vi "Autunomous Set Target.vi"() -> ()   [LabVIEW 2009]
uses:
  <vilib>/Platform/TimedLoop/XDataNode/XDataNode.xnode
  <vilib>/Platform/TimedLoop/XDataNode/loadlvalarms.vi
  <vilib>/Platform/TimedLoop/XDataNode/timing_clust.ctl
  <vilib>/Platform/TimedLoop/XDataNode/nitl_modes.ctl
  <vilib>/Platform/TimedLoop/XDataNode/wakeup.ctl
  TypeDefs/State Machine/Main State.ctl
  Functional Global Variables/Actions for FG's.ctl
  TypeDefs/Sensor TypeDefs/GPS Data.ctl
  <vilib>/Platform/TimedLoop/XDataNode/XDNodeRunTimeDep.lvlib
  <vilib>/Analysis/NI_AALBase.lvlib
  <vilib>/Analysis/NI_AALPro.lvlib
panel:
  in  "Buffer Size (Seconds)":i32=15
  in  "Path history enabled?":bool=TRUE
  in  "Buffer Dimension":i32=10
  out "Target Bearing":dbl
  in  "Prediction Time (s)":dbl=1.0
  out "XY Graph":cluster{dbl[], dbl[]}(graph)
  in  "Sampling Time":dbl[](array[numeric])
  in  "Bearing History":dbl[](array[numeric])
  out "Bearing Sample":dbl=191.29579607174375 format="%0.2f"
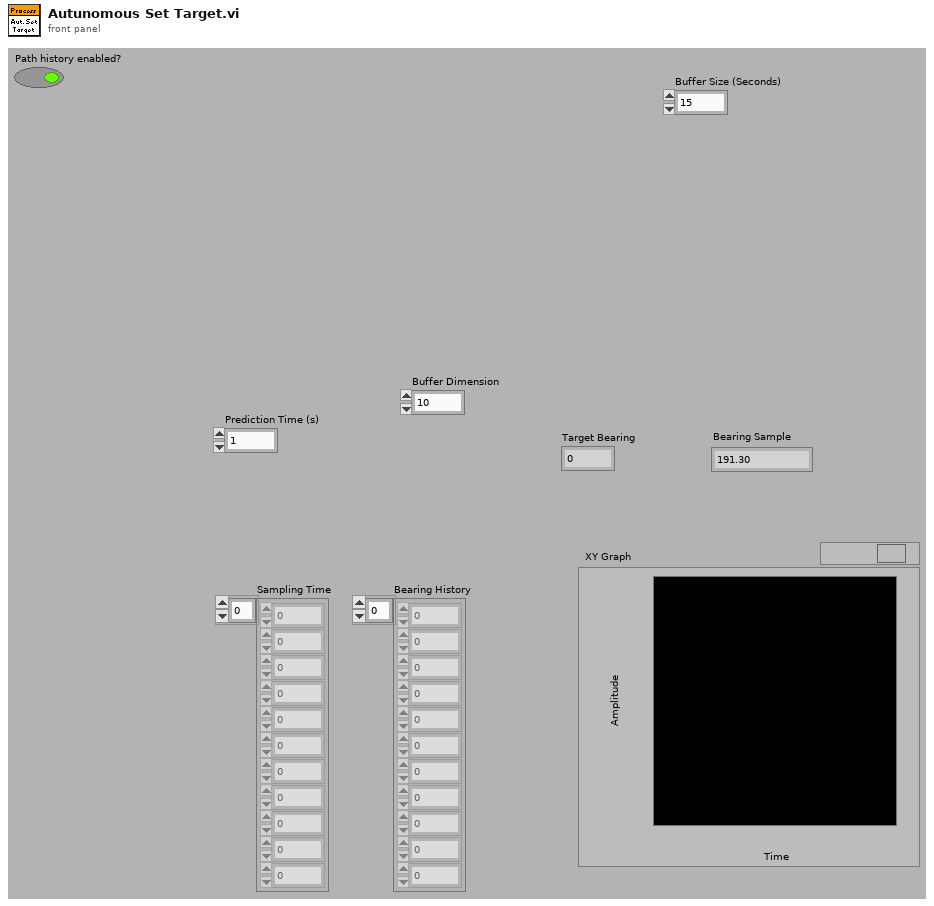
[diagram p1: front panel]
types:
  T1 = typedef "Actions for FG's.ctl" = enum16{"Read", "Write"}
  T2 = typedef "XDNodeRunTimeDep.lvlib/timing_clust.ctl" = cluster{"Expected End [f-1]":u64, "Actual End [f-1]":u64, "Finished Late? [f-1]":bool, "Expected End [i-1]":u64, "Actual End [i-1]":u64, "Finished Late? [i-1]":bool, "Expected Start [i]":u64, "Actual Start [i]":u64, "Expected Start [f]":u64, "Actual Start [f]":u64, "Source Name":string, "Structure Name":string, "Period":i64, "Deadline":i64, "Offset":i64, "Start":i64, "Priority":i32, "Timeout":i32, "Mode":T3, "Wakeup Reason":T4, "Error":errorcluster, "Source Type":string, "Secondary Source Type":string, "Global End Time":u64, "Global Start Time":u64, "Frame Duration":u64, "Iteration Duration":u64, "Assigned CPU":i32, "I/O Scan Engine Mode":u32}
  T3 = typedef "XDNodeRunTimeDep.lvlib/nitl_modes.ctl" = enum32{"No Change", "Process missed periods, maintain original phase", "Discard missed periods, maintain original phase", "Process missed periods, ignore original phase", "Discard missed periods, ignore original phase"}
  T4 = typedef "XDNodeRunTimeDep.lvlib/wakeup.ctl" = enum32{"Normal", "Aborted", "Asynchronous wakeup", "Timing source error", "Timed loop error", "Timeout"}
  T5 = typedef "Main State.ctl" = enum16{"Startup", "Wait for Init", "Initialize Sensors", "Wait for Saftey Disable", "Check Saftey", "Wait for GO", "Run", "Remote Control", "Stop"}
  T6 = typedef "GPS Data.ctl" = cluster{"Latitude":dbl, "Longitude":dbl}
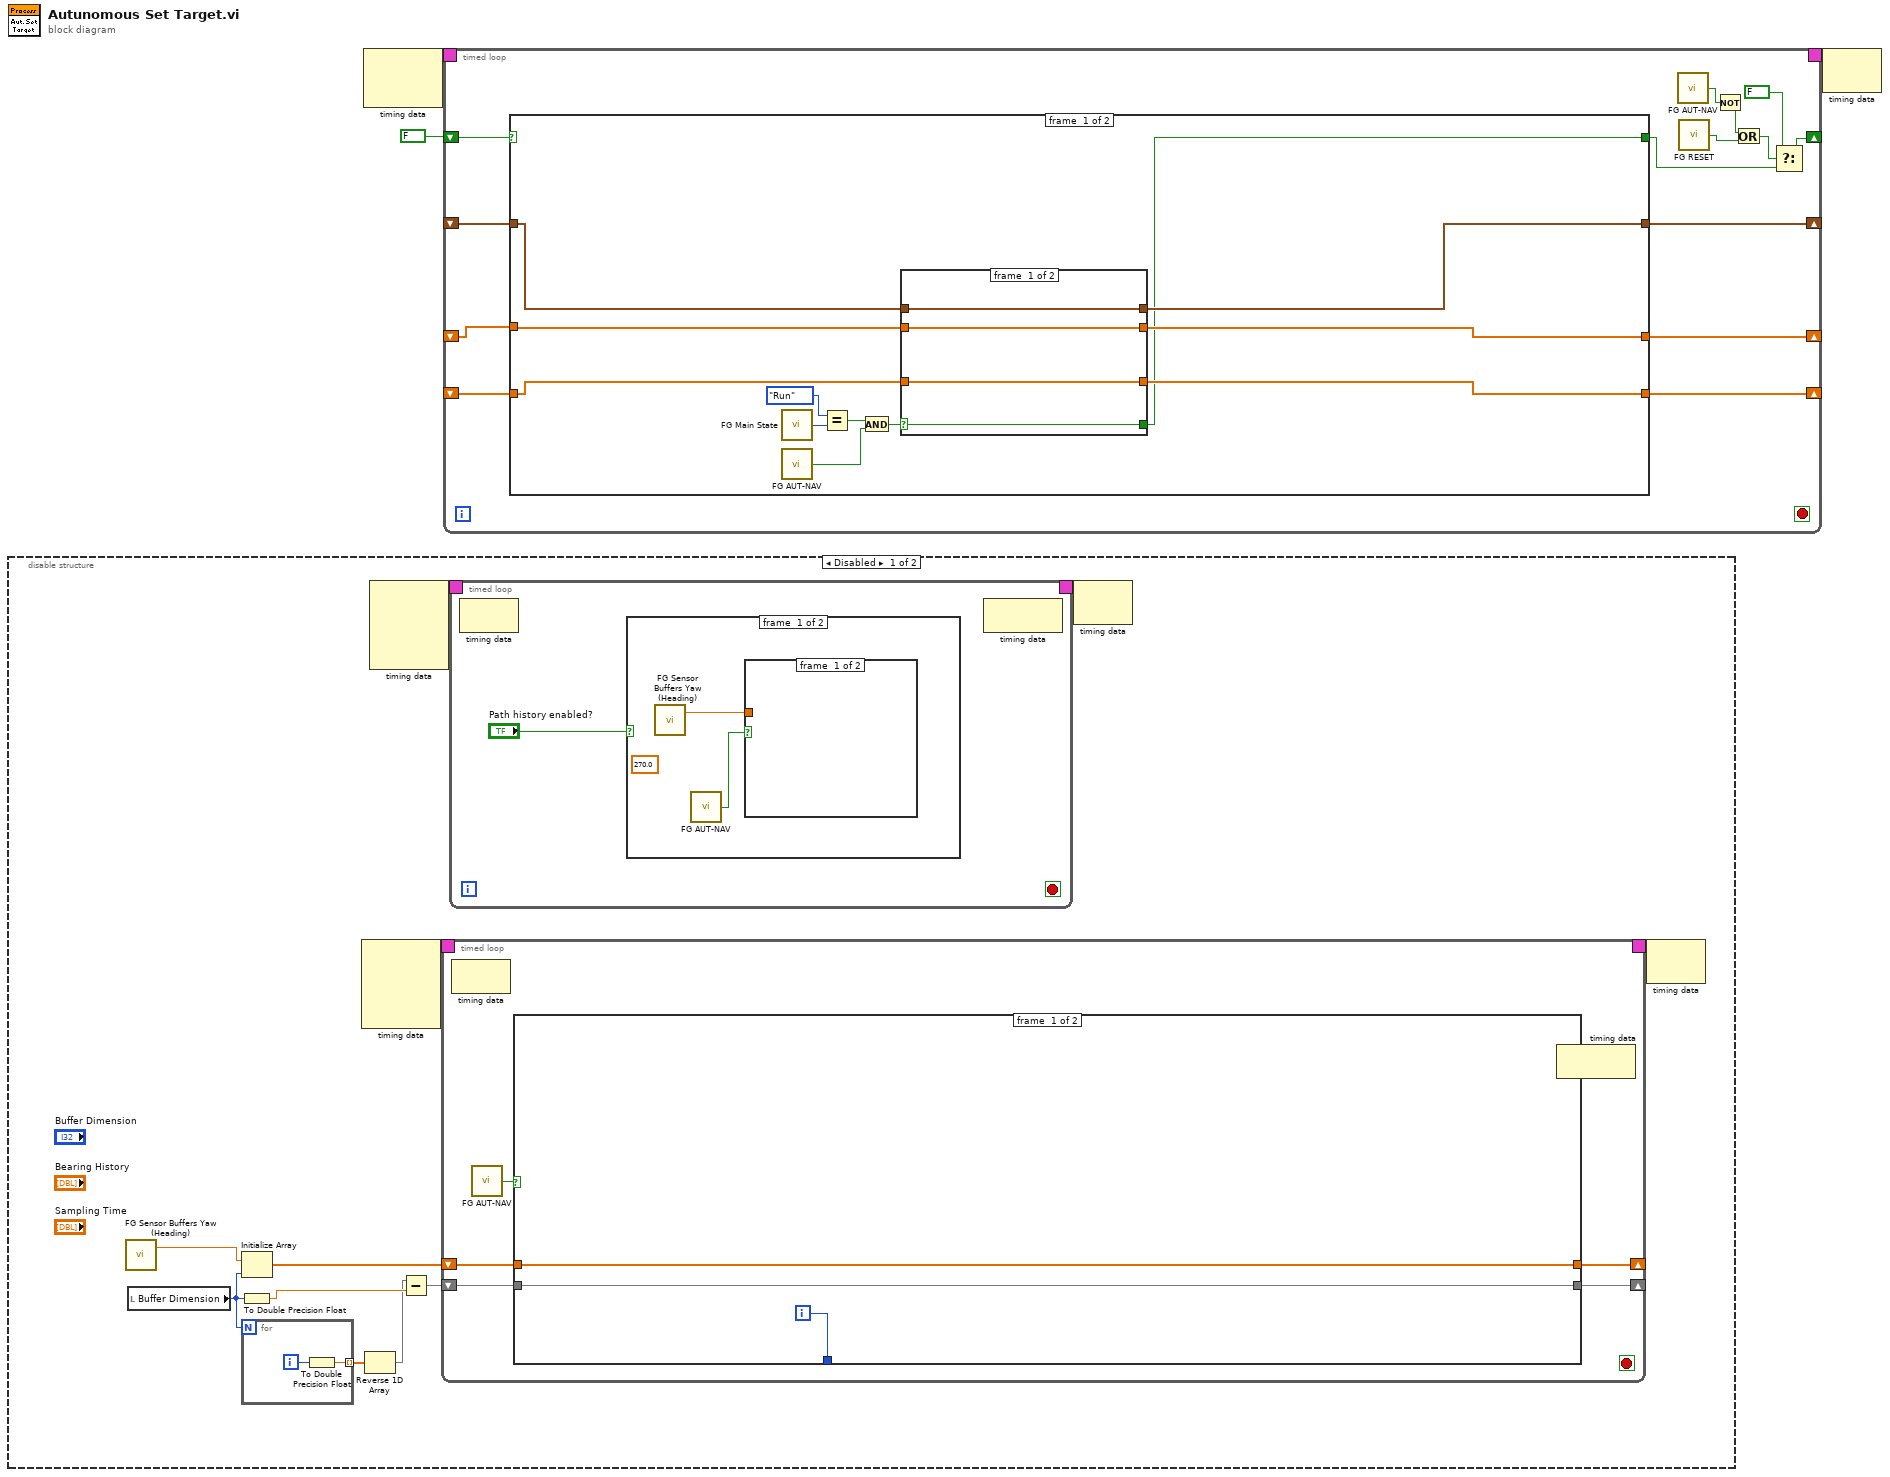
[diagram p0: block diagram]
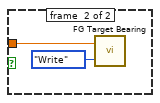
[diagram p2: hidden frame]
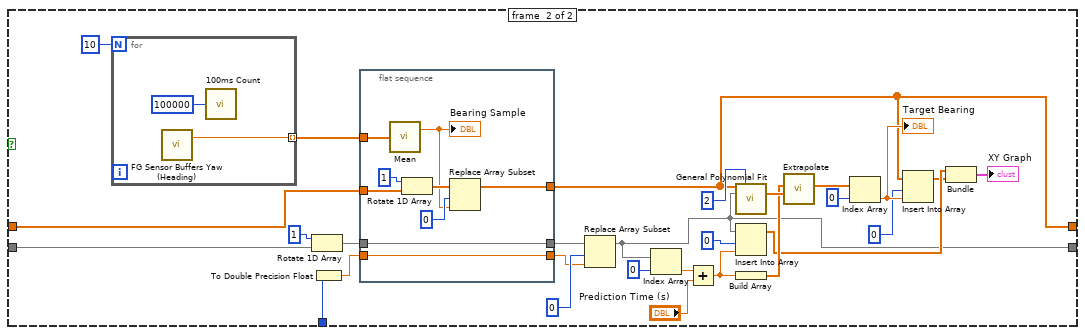
[diagram p4: hidden frame]
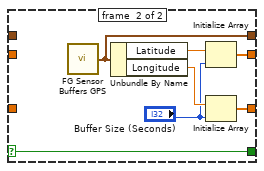
[diagram p6: hidden frame]
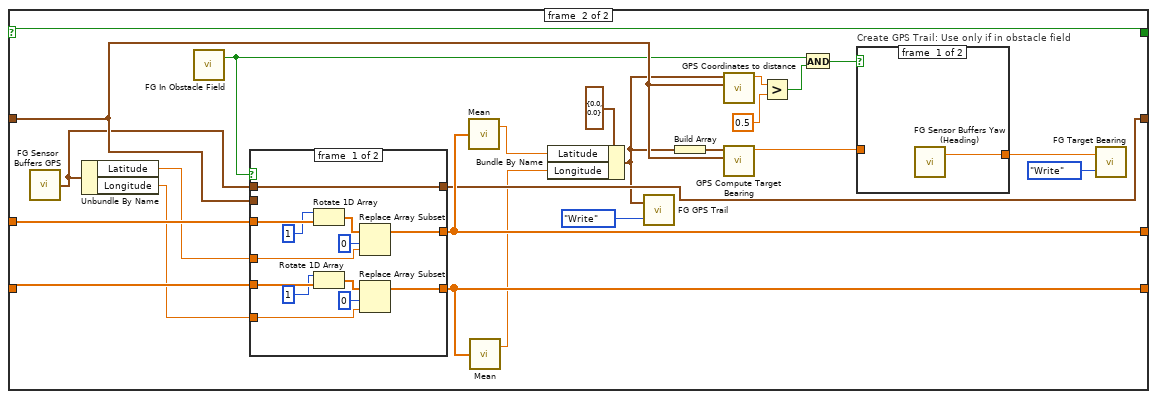
[diagram p7: hidden frame]
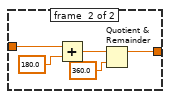
[diagram p8: hidden frame]
diagram:
  n1 = disable-structure shown="Disabled" {
    frame #0 {
      n2 = call "FG Sensor Buffers Yaw (Heading).vi"() -> ("Yaw Buffer Out"=w10:dbl)  [unwired: 3 in]
      n3 = local read "Buffer Dimension"() -> (w7:i32)
      n4 = Initialize Array(w10, w7) -> (w9:dbl[])
      n5 = To Double Precision Float(number=w7) -> (double precision float=w5:dbl)
      n6 = for {
        N: w7 -> [_]
        tunnel: [w24] -> w8 mode=indexing
        i -> [w25]
        n7 = To Double Precision Float(number=w25) -> (double precision float=w24:dbl)
      }
      n8 = node-c288() -> (w14:T2)  [unwired: 4 in]
      n9 = Reverse 1D Array(array=w8) -> (reversed array=w4:dbl[])
      n10 = node-c288() -> (w12:T2)  [unwired: 4 in]
      n11 = Subtract(x=w4, y=w5) -> (x-y=w6:dbl[])
      n12 = timed-loop {
        timing: w14 -> [_]
        timing-out: [_] -> w13
        shift-right: [w28] -> _
        shift-left: w9 -> [w29]
        shift-right: [w27] -> _
        shift-left: w6 -> [w30]
        i -> [w31]
        stop <- _ stop-if-true
        n13 = node-c288() -> ()  [unwired: 1 in, 1 out]
        n14 = call "FG AUT-NAV.vi"() -> ("Aut/!Nav out"=w26:bool)  [unwired: 2 in]
        n15 = case shown="True" w26 {
          tunnel: w31 -> [_ w59]
          tunnel: w30 -> [w32 w58]
          tunnel: w29 -> [w33 w51]
          tunnel: [w33 w35] -> w28
          tunnel: [w32 w34] -> w27
          frame #0 {
          }
          frame #1 {
            n16 = for {
              N: 10 -> [_]
              tunnel: [w72] -> w60 mode=indexing
              n17 = call "FG Sensor Buffers Yaw (Heading).vi"() -> ("Yaw Buffer Out"=w72:dbl)  [unwired: 3 in]
              n18 = call "100ms Count"("Count(uSec)"=u32 100000) -> ()  [unwired: 1 out]
            }
            n19 = Rotate 1D Array(1:w58, 2:1 ("n")) -> (0:w56:dbl[])
            n20 = To Double Precision Float(number=w59) -> (double precision float=w55:dbl)
            n21 = flat-sequence {
              tunnel: w60 -> [w70]
              tunnel: w56 -> [w69]
              tunnel: w55 -> [w68]
              tunnel: [w69] -> w53
              tunnel: [w68] -> w52
              tunnel: w51 -> [w66]
              tunnel: [w63] -> w35
              frame #0 {
                n22 = call <vilib>:"Mean.vi"("X"=w70) -> ("mean"=w62:dbl)  [unwired: 1 out]
                "Bearing Sample" <- w62
                n23 = Rotate 1D Array(1:w66, 2:1 ("n")) -> (0:w64:dbl[])
                n24 = Replace Array Subset(array=w64, new element=w62, index=0) -> (w63:dbl[])
              }
            }
            n25 = Replace Array Subset(array=w53, new element=w52, index=0) -> (w34:dbl[])
            n26 = Index Array(array=w34, index=0) -> (element=w46:dbl)
            n27 = Add(x=w46, y="Prediction Time (s)") -> (x+y=w40:dbl)
            n28 = call <vilib>:"General Polynomial Fit.vi"("Y"=w35, "polynomial order"=2, "X"=w34) -> ("Polynomial Coefficients"=w49:dbl[])  [unwired: 9 in, 3 out]
            n29 = Insert Into Array(array=w34, index=0, new element=w40) -> (w39:dbl[])
            n30 = Build Array(w40) -> (w41:dbl[])
            n31 = call "Extrapolate.vi"("Polynomial Coefficients"=w49, "xi"=w41) -> ("yi"=w48:dbl[])  [unwired: 9 in]
            n32 = Index Array(array=w48, index=0) -> (element=w42:dbl)
            "Target Bearing" <- w42
            n33 = Insert Into Array(array=w35, index=0, new element=w42) -> (w38:dbl[])
            n34 = Bundle(w39, w38) -> (→"XY Graph":cluster{dbl[], dbl[]})  [unwired: 1 in]
          }
        }
        n35 = node-c288() -> ()  [unwired: 1 in, 1 out]
      }
      n36 = timed-loop {
        timing: w12 -> [_]
        timing-out: [_] -> w11
        stop <- _ stop-if-true
        n37 = node-c288() -> ()  [unwired: 1 in, 1 out]
        n38 = case shown="False" "Path history enabled?" {
          frame #0 {
            (unwired) 270.0 ("Target Bearing in")
            n39 = call "FG Sensor Buffers Yaw (Heading).vi"() -> ("Yaw Buffer Out"=w17:dbl)  [unwired: 3 in]
            n40 = call "FG AUT-NAV.vi"() -> ("Aut/!Nav out"=w16:bool)  [unwired: 2 in]
            n41 = case shown="True" w16 {
              tunnel: w17 -> [_ w18]
              frame #0 {
              }
              frame #1 {
                n42 = call "FG Target Bearing.vi"("FG Action (Read)"=Actions_for_FG's."Write", "Target Bearing in"=w18) -> ()  [unwired: 1 out]
              }
            }
          }
          frame #1 {
          }
        }
        n43 = node-c288() -> ()  [unwired: 1 in, 1 out]
      }
      n44 = node-c288(w11) -> ()  [unwired: 1 out]
      n45 = node-c288(w13) -> ()  [unwired: 1 out]
    }
    frame #1 {
    }
  }
  n46 = node-c288() -> (w3:T2)  [unwired: 2 in]
  n47 = timed-loop {
    timing: w3 -> [_]
    timing-out: [_] -> w2
    shift-right: [w88] -> _
    shift-left: _ -> [w90]
    shift-right: [w87] -> _
    shift-left: _ -> [w89]
    shift-right: [w85] -> _
    shift-left: _ -> [w86]
    shift-right: [w82] -> _
    shift-left: FALSE ("t") -> [w84]
    stop <- _ stop-if-true
    n48 = case shown="False" w84 {
      selector: w84 -> [_ w115]
      tunnel: w90 -> [w93 w137]
      tunnel: w89 -> [w92 w136]
      tunnel: [w97 w135] -> w88
      tunnel: [w96 w134] -> w87
      tunnel: w86 -> [w94 w133]
      tunnel: [w95 w132] -> w85
      tunnel: [w91 w115] -> w81
      frame #0 {
        n49 = call "FG Main State.vi"() -> ("Main State out"=w102:T5)  [unwired: 2 in]
        n50 = call "FG AUT-NAV.vi"() -> ("Aut/!Nav out"=w98:bool)  [unwired: 2 in]
        n51 = Equal?(x=Main_State."Run" ("Main State out"), y=w102) -> (x = y?=w100:bool)
        n52 = And(x=w100, y=w98) -> (x .and. y?=w99:bool)
        n53 = case shown="False" w99 {
          selector: w99 -> [w103 w108]
          tunnel: [w105 w111] -> w97
          tunnel: [w104 w110] -> w96
          tunnel: [w106 w109] -> w95
          tunnel: w94 -> [w106 _]
          tunnel: w93 -> [w105 _]
          tunnel: w92 -> [w104 _]
          tunnel: [w103 w108] -> w91
          frame #0 {
          }
          frame #1 {
            n54 = call "FG Sensor Buffers GPS.vi"() -> ("GPS Buffer out"=w109:T6)  [unwired: 2 in]
            n55 = Unbundle By Name(w109) -> ("Latitude"=w112:dbl, "Longitude"=w113:dbl)
            n56 = Initialize Array(w112, "Buffer Size (Seconds)") -> (w111:dbl[])
            n57 = Initialize Array(w113, "Buffer Size (Seconds)") -> (w110:dbl[])
          }
        }
      }
      frame #1 {
        n58 = call "FG Sensor Buffers GPS.vi"() -> ("GPS Buffer out"=w123:T6)  [unwired: 2 in]
        n59 = Unbundle By Name(w123) -> ("Latitude"=w131:dbl, "Longitude"=w130:dbl)
        n60 = call "FG In Obstacle Field.vi"() -> ("In Obs. Field? out"=w116:bool)  [unwired: 3 in]
        n61 = case shown="False" w116 {
          tunnel: w137 -> [w156 w158]
          tunnel: w136 -> [w155 w157]
          tunnel: w131 -> [w154 _]
          tunnel: w130 -> [w153 _]
          tunnel: [w146 w158] -> w135
          tunnel: [w145 w157] -> w134
          tunnel: w123 -> [w144 _]
          tunnel: [w144 w159] -> w132
          tunnel: w133 -> [_ w159]
          frame #0 {
            n62 = Rotate 1D Array(1:w156, 2:1 ("n")) -> (0:w150:dbl[])
            n63 = Rotate 1D Array(1:w155, 2:1 ("n")) -> (0:w149:dbl[])
            n64 = Replace Array Subset(array=w150, new element=w154, index=0) -> (w146:dbl[])
            n65 = Replace Array Subset(array=w149, new element=w153, index=0) -> (w145:dbl[])
          }
          frame #1 {
          }
        }
        n66 = call <vilib>:"Mean.vi"("X"=w135) -> ("mean"=w128:dbl)  [unwired: 1 out]
        n67 = call <vilib>:"Mean.vi"("X"=w134) -> ("mean"=w124:dbl)  [unwired: 1 out]
        n68 = Bundle By Name(cluster=T6 {"Latitude"=0.0, "Longitude"=0.0} ("GPS Buffer out"), "Latitude"=w128, "Longitude"=w124) -> (w119:T6)
        n69 = call "FG GPS Trail.vi"("FG Action (Read)"=Actions_for_FG's."Write", "GPS Buffer in"=w119) -> ()  [unwired: 1 in, 1 out]
        n70 = Build Array(w119) -> (w126:T6[])
        n71 = call "GPS Coordinates to distance.vi"("GPS Co-ordinate 2"=w133, "GPS Co-ordinate 1"=w119) -> ("Distance"=w118:dbl)  [unwired: 9 in]
        n72 = call "GPS Compute Target Bearing.vi"("Current co-ordinates"=w133, "GPS Waypoint List Out"=w126) -> ("Target Bearing (degrees)"=w125:dbl)  [unwired: 8 in]
        n73 = Greater?(x=w118, y=0.5) -> (0:w120:bool)
        n74 = And(x=w116, y=w120) -> (x .and. y?=w114:bool)
        n75 = case "Create GPS Trail: Use only if in obstacle field" shown="True" w114 {
          tunnel: w125 -> [_ w143]
          tunnel: [w138 w142] -> w121
          frame #0 {
            n76 = call "FG Sensor Buffers Yaw (Heading).vi"() -> ("Yaw Buffer Out"=w138:dbl)  [unwired: 3 in]
          }
          frame #1 {
            n77 = Add(x=w143, y=180.0) -> (x+y=w140:dbl)
            n78 = Quotient & Remainder(x=w140, y=360.0) -> (x-y*floor(x/y)=w142:dbl)  [unwired: 1 out]
          }
        }
        n79 = call "FG Target Bearing.vi"("FG Action (Read)"=Actions_for_FG's."Write", "Target Bearing in"=w121) -> ()  [unwired: 1 out]
      }
    }
    n80 = call "FG AUT-NAV.vi"() -> ("Aut/!Nav out"=w80:bool)  [unwired: 2 in]
    n81 = call "FG RESET.vi"() -> ("RESET out"=w78:bool)  [unwired: 2 in]
    n82 = Not(x=w80) -> (.not. x?=w79:bool)
    n83 = Or(x=w79, y=w78) -> (x .or. y?=w77:bool)
    n84 = Select(t=FALSE, s=w77, f=w81) -> (s? t:f=w82:bool)
  }
  n85 = node-c288(w2) -> ()  [unwired: 1 out]
